vi "Starts With.vi"() -> ()   [LabVIEW 2017, in "Assertions.Tests.lvlib" / "Assert String Starts With.lvlib"]
uses:
  Assert String Starts With.lvlib
  src/Transparent Assertions/Assertions/Assertions.lvlib
panel:
  out "error out":errorcluster
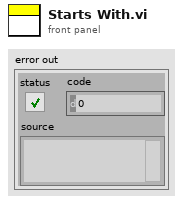
[diagram p1: front panel]
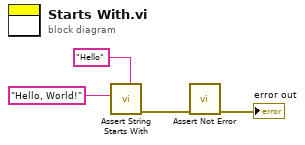
[diagram p0: block diagram]
diagram:
  n1 = call "Assert String Starts With.vi"("Prefix"="Hello", "String"="Hello, World!") -> ("error out"=w2:errorcluster)  [unwired: 9 in]
  n2 = call "Assert Not Error.vi"("error in (no error)"=w2) -> ("error out"=→"error out":errorcluster)  [unwired: 10 in]
